vi "FTW-Request-Construct.vi"(5 "Server Address":string, 11 "error in":errorcluster) -> (4 "FTW-Request Out":refnum<class "FTW-Request.lvclass">, 15 "error out":errorcluster)   [LabVIEW 2015, in "FTW-Request.lvclass"]
uses:
  FTW-Request.lvclass
  Ether/FTW-Ether-EndpointType.ctl
  FTW-Request.lvclass/FTW-Request.ctl
  Endpoint/FTW-Endpoint.lvclass
  Ether/FTW-Ether.lvclass
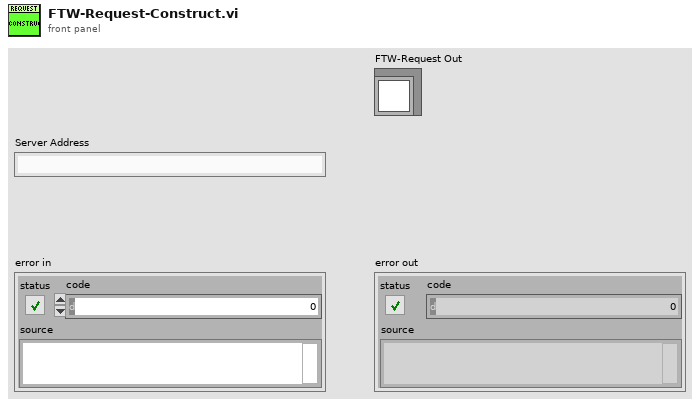
[diagram p1: front panel]
types:
  T1 = typedef "FTW-Ether.lvclass/FTW-Ether-EndpointType.ctl" = enum16{"Server", "Client", "Publisher", "Subscriber"}
  T2 = typedef "FTW-Ether.lvclass/FTW-Ether-MessageTransportScheme.ctl" = enum16{"In process (inproc://)", "TCP (tcp://)"}
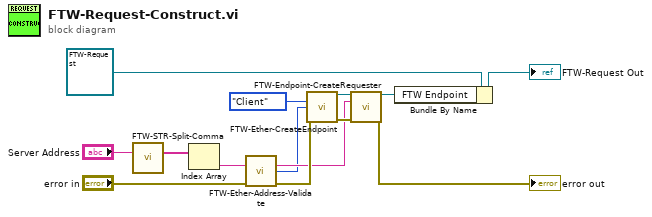
[diagram p0: block diagram]
diagram:
  n1 = call "FTW-STR-Split-Comma.vi"("Delimited String"="Server Address") -> ("Array of Strings"=w2:string[])  [unwired: 14 in]
  n2 = Index Array(array=w2) -> (element=w1:string)  [unwired: 1 in]
  n3 = call "FTW-Ether-Address-Validate.vi"("Address"=w1, "error in"="error in") -> ("Sanitized Address"=w5:string, "Message Transport Scheme"=w4:T2, "error out"=w9:errorcluster)  [unwired: 11 in]
  n4 = call "FTW-Ether-CreateEndpoint.vi"("Endpoint Type"=FTW-Ether-EndpointType."Client", "Message Transport Scheme"=w4, "error in"=w9) -> ("FTW Endpoint"=w6:refnum<class "FTW-Endpoint.lvclass">, "error out"=w7:errorcluster)  [unwired: 11 in]
  n5 = call-dynamic "FTW-Endpoint-CreateRequester.vi"("FTW Endpoint"=w6, "Endpoint Address"=w5, "error in"=w7) -> ("FTW Endpoint out"=w3:refnum<class "FTW-Endpoint.lvclass">, "error out"=→"error out":errorcluster)  [unwired: 11 in]
  n6 = Bundle By Name(cluster=refnum<class "FTW-Request.lvclass"> refnum ("LVmsg_Client in"), "FTW Endpoint"=w3) -> (→"FTW-Request Out":refnum<class "FTW-Request.lvclass">)
